vi "Main.vi"() -> ()   [LabVIEW 2015]
panel:
  in  "Load Config":bool
  in  "Save Config":bool
  in  "Configuation Path":path
  out "Real Milliseconds per Packet":sgl=50.0
  in  "Apply New Milliseconds":bool
  in  "Milliseconds per Packet":sgl=50.0
  in  "Apply New X Axis":bool
  in  "Number of Seconds Visible":dbl=10.0
  in  "0":T1={"DeviceType"=0, "DeviceID"=0, "PropertyID"=0, "UpdateProperty"=FALSE, "Current Value"=0.0, "Y-Axis"=0, "Plot Color"=16777215, "Point Color"=16777216} {"DeviceType" items=["Talon", "DIO", "RoboRIO"]; "Y-Axis" items=["Red Axis", "Blue Axis", "Green Axis", "Yellow Axis"]}
  in  "Plot":T2={"0"={"DeviceType"=0, "DeviceID"=0, "PropertyID"=0, "UpdateProperty"=FALSE, "Current Value"=0.0, "Y-Axis"=0, "Plot Color"=16777215, "Point Color"=16777216}, "0 2"={"DeviceType"=0, "DeviceID"=0, "PropertyID"=0, "UpdateProperty"=FALSE, "Current Value"=0.0, "Y-Axis"=0, "Plot Color"=16777215, "Point Color"=16777216}, "0 3"={"DeviceType"=0, "DeviceID"=0, "PropertyID"=0, "UpdateProperty"=FALSE, "Current Value"=0.0, "Y-Axis"=0, "Plot Color"=16777215, "Point Color"=16777216}, "0 4"={"DeviceType"=0, "DeviceID"=0, "PropertyID"=0, "UpdateProperty"=FALSE, "Current Value"=0.0, "Y-Axis"=0, "Plot Color"=16777215, "Point Color"=16777216}, "0 5"={"DeviceType"=0, "DeviceID"=0, "PropertyID"=0, "UpdateProperty"=FALSE, "Current Value"=0.0, "Y-Axis"=0, "Plot Color"=16777215, "Point Color"=16777216}, "0 6"={"DeviceType"=0, "DeviceID"=0, "PropertyID"=0, "UpdateProperty"=FALSE, "Current Value"=0.0, "Y-Axis"=0, "Plot Color"=16777215, "Point Color"=16777216}, "0 7"={"DeviceType"=0, "DeviceID"=0, "PropertyID"=0, "UpdateProperty"=FALSE, "Current Value"=0.0, "Y-Axis"=0, "Plot Color"=16777215, "Point Color"=16777216}, "0 8"={"DeviceType"=0, "DeviceID"=0, "PropertyID"=0, "UpdateProperty"=FALSE, "Current Value"=0.0, "Y-Axis"=0, "Plot Color"=16777215, "Point Color"=16777216}, "0 9"={"DeviceType"=0, "DeviceID"=0, "PropertyID"=0, "UpdateProperty"=FALSE, "Current Value"=0.0, "Y-Axis"=0, "Plot Color"=16777215, "Point Color"=16777216}, "0 10"={"DeviceType"=0, "DeviceID"=0, "PropertyID"=0, "UpdateProperty"=FALSE, "Current Value"=0.0, "Y-Axis"=0, "Plot Color"=16777215, "Point Color"=16777216}, "0 11"={"DeviceType"=0, "DeviceID"=0, "PropertyID"=0, "UpdateProperty"=FALSE, "Current Value"=0.0, "Y-Axis"=0, "Plot Color"=16777215, "Point Color"=16777216}, "0 12"={"DeviceType"=0, "DeviceID"=0, "PropertyID"=0, "UpdateProperty"=FALSE, "Current Value"=0.0, "Y-Axis"=0, "Plot Color"=16777215, "Point Color"=16777216}, "0 13"={"DeviceType"=0, "DeviceID"=0, "PropertyID"=0, "UpdateProperty"=FALSE, "Current Value"=0.0, "Y-Axis"=0, "Plot Color"=16777215, "Point Color"=16777216}, "0 14"={"DeviceType"=0, "DeviceID"=0, "PropertyID"=0, "UpdateProperty"=FALSE, "Current Value"=0.0, "Y-Axis"=0, "Plot Color"=16777215, "Point Color"=16777216}, "0 15"={"DeviceType"=0, "DeviceID"=0, "PropertyID"=0, "UpdateProperty"=FALSE, "Current Value"=0.0, "Y-Axis"=0, "Plot Color"=16777215, "Point Color"=16777216}, "0 16"={"DeviceType"=0, "DeviceID"=0, "PropertyID"=0, "UpdateProperty"=FALSE, "Current Value"=0.0, "Y-Axis"=0, "Plot Color"=16777215, "Point Color"=16777216}} {"0 16"."DeviceID" items=["2"]; "0 16"."PropertyID" items=["SetValue", "OutputVoltage", "OutputCurrent", "EncoderPosition", "EncoderVelocity", "CTR_Absolute_Pos", "ControlLoop_Error", "I Accum", "Supply Voltage", "Forward Hard Limit", "Reverse Hard Limit", "Forward Soft Limit", "Reverse Soft Limit", "Analog In"]; "0 16"."DeviceType" items=["Talon", "DIO", "RoboRIO"]; "0 16"."Y-Axis" items=["Red Axis", "Blue Axis", "Green Axis", "Yellow Axis"]; "0 15"."DeviceID" items=["2"]; "0 15"."PropertyID" items=["SetValue", "OutputVoltage", "OutputCurrent", "EncoderPosition", "EncoderVelocity", "CTR_Absolute_Pos", "ControlLoop_Error", "I Accum", "Supply Voltage", "Forward Hard Limit", "Reverse Hard Limit", "Forward Soft Limit", "Reverse Soft Limit", "Analog In"]; "0 15"."DeviceType" items=["Talon", "DIO", "RoboRIO"]; "0 15"."Y-Axis" items=["Red Axis", "Blue Axis", "Green Axis", "Yellow Axis"]; "0 14"."DeviceID" items=["2"]; "0 14"."PropertyID" items=["SetValue", "OutputVoltage", "OutputCurrent", "EncoderPosition", "EncoderVelocity", "CTR_Absolute_Pos", "ControlLoop_Error", "I Accum", "Supply Voltage", "Forward Hard Limit", "Reverse Hard Limit", "Forward Soft Limit", "Reverse Soft Limit", "Analog In"]; "0 14"."DeviceType" items=["Talon", "DIO", "RoboRIO"]; "0 14"."Y-Axis" items=["Red Axis", "Blue Axis", "Green Axis", "Yellow Axis"]; "0 13"."DeviceID" items=["2"]; "0 13"."PropertyID" items=["SetValue", "OutputVoltage", "OutputCurrent", "EncoderPosition", "EncoderVelocity", "CTR_Absolute_Pos", "ControlLoop_Error", "I Accum", "Supply Voltage", "Forward Hard Limit", "Reverse Hard Limit", "Forward Soft Limit", "Reverse Soft Limit", "Analog In"]; "0 13"."DeviceType" items=["Talon", "DIO", "RoboRIO"]; "0 13"."Y-Axis" items=["Red Axis", "Blue Axis", "Green Axis", "Yellow Axis"]; "0 12"."DeviceID" items=["2"]; "0 12"."PropertyID" items=["SetValue", "OutputVoltage", "OutputCurrent", "EncoderPosition", "EncoderVelocity", "CTR_Absolute_Pos", "ControlLoop_Error", "I Accum", "Supply Voltage", "Forward Hard Limit", "Reverse Hard Limit", "Forward Soft Limit", "Reverse Soft Limit", "Analog In"]; "0 12"."DeviceType" items=["Talon", "DIO", "RoboRIO"]; "0 12"."Y-Axis" items=["Red Axis", "Blue Axis", "Green Axis", "Yellow Axis"]; "0 11"."DeviceID" items=["2"]; "0 11"."PropertyID" items=["SetValue", "OutputVoltage", "OutputCurrent", "EncoderPosition", "EncoderVelocity", "CTR_Absolute_Pos", "ControlLoop_Error", "I Accum", "Supply Voltage", "Forward Hard Limit", "Reverse Hard Limit", "Forward Soft Limit", "Reverse Soft Limit", "Analog In"]; "0 11"."DeviceType" items=["Talon", "DIO", "RoboRIO"]; "0 11"."Y-Axis" items=["Red Axis", "Blue Axis", "Green Axis", "Yellow Axis"]; "0 10"."DeviceID" items=["2"]; "0 10"."PropertyID" items=["SetValue", "OutputVoltage", "OutputCurrent", "EncoderPosition", "EncoderVelocity", "CTR_Absolute_Pos", "ControlLoop_Error", "I Accum", "Supply Voltage", "Forward Hard Limit", "Reverse Hard Limit", "Forward Soft Limit", "Reverse Soft Limit", "Analog In"]; "0 10"."DeviceType" items=["Talon", "DIO", "RoboRIO"]; "0 10"."Y-Axis" items=["Red Axis", "Blue Axis", "Green Axis", "Yellow Axis"]; "0 9"."DeviceID" items=["2"]; "0 9"."PropertyID" items=["SetValue", "OutputVoltage", "OutputCurrent", "EncoderPosition", "EncoderVelocity", "CTR_Absolute_Pos", "ControlLoop_Error", "I Accum", "Supply Voltage", "Forward Hard Limit", "Reverse Hard Limit", "Forward Soft Limit", "Reverse Soft Limit", "Analog In"]; "0 9"."DeviceType" items=["Talon", "DIO", "RoboRIO"]; "0 9"."Y-Axis" items=["Red Axis", "Blue Axis", "Green Axis", "Yellow Axis"]; "0 8"."DeviceID" items=["2"]; "0 8"."PropertyID" items=["SetValue", "OutputVoltage", "OutputCurrent", "EncoderPosition", "EncoderVelocity", "CTR_Absolute_Pos", "ControlLoop_Error", "I Accum", "Supply Voltage", "Forward Hard Limit", "Reverse Hard Limit", "Forward Soft Limit", "Reverse Soft Limit", "Analog In"]; "0 8"."DeviceType" items=["Talon", "DIO", "RoboRIO"]; "0 8"."Y-Axis" items=["Red Axis", "Blue Axis", "Green Axis", "Yellow Axis"]; "0 7"."DeviceID" items=["2"]; "0 7"."PropertyID" items=["SetValue", "OutputVoltage", "OutputCurrent", "EncoderPosition", "EncoderVelocity", "CTR_Absolute_Pos", "ControlLoop_Error", "I Accum", "Supply Voltage", "Forward Hard Limit", "Reverse Hard Limit", "Forward Soft Limit", "Reverse Soft Limit", "Analog In"]; "0 7"."DeviceType" items=["Talon", "DIO", "RoboRIO"]; "0 7"."Y-Axis" items=["Red Axis", "Blue Axis", "Green Axis", "Yellow Axis"]; "0 6"."DeviceID" items=["2"]; "0 6"."PropertyID" items=["SetValue", "OutputVoltage", "OutputCurrent", "EncoderPosition", "EncoderVelocity", "CTR_Absolute_Pos", "ControlLoop_Error", "I Accum", "Supply Voltage", "Forward Hard Limit", "Reverse Hard Limit", "Forward Soft Limit", "Reverse Soft Limit", "Analog In"]; "0 6"."DeviceType" items=["Talon", "DIO", "RoboRIO"]; "0 6"."Y-Axis" items=["Red Axis", "Blue Axis", "Green Axis", "Yellow Axis"]; "0 5"."DeviceID" items=["2"]; "0 5"."PropertyID" items=["SetValue", "OutputVoltage", "OutputCurrent", "EncoderPosition", "EncoderVelocity", "CTR_Absolute_Pos", "ControlLoop_Error", "I Accum", "Supply Voltage", "Forward Hard Limit", "Reverse Hard Limit", "Forward Soft Limit", "Reverse Soft Limit", "Analog In"]; "0 5"."DeviceType" items=["Talon", "DIO", "RoboRIO"]; "0 5"."Y-Axis" items=["Red Axis", "Blue Axis", "Green Axis", "Yellow Axis"]; "0 4"."DeviceID" items=["2"]; "0 4"."PropertyID" items=["SetValue", "OutputVoltage", "OutputCurrent", "EncoderPosition", "EncoderVelocity", "CTR_Absolute_Pos", "ControlLoop_Error", "I Accum", "Supply Voltage", "Forward Hard Limit", "Reverse Hard Limit", "Forward Soft Limit", "Reverse Soft Limit", "Analog In"]; "0 4"."DeviceType" items=["Talon", "DIO", "RoboRIO"]; "0 4"."Y-Axis" items=["Red Axis", "Blue Axis", "Green Axis", "Yellow Axis"]; "0 3"."DeviceID" items=["2"]; "0 3"."PropertyID" items=["SetValue", "OutputVoltage", "OutputCurrent", "EncoderPosition", "EncoderVelocity", "CTR_Absolute_Pos", "ControlLoop_Error", "I Accum", "Supply Voltage", "Forward Hard Limit", "Reverse Hard Limit", "Forward Soft Limit", "Reverse Soft Limit", "Analog In"]; "0 3"."DeviceType" items=["Talon", "DIO", "RoboRIO"]; "0 3"."Y-Axis" items=["Red Axis", "Blue Axis", "Green Axis", "Yellow Axis"]; "0 2"."DeviceID" items=["0"]; "0 2"."PropertyID" items=["PacketCounter", "Milliseconds Per Packet", "CPU Load"]; "0 2"."DeviceType" items=["Talon", "DIO", "RoboRIO"]; "0 2"."Y-Axis" items=["Red Axis", "Blue Axis", "Green Axis", "Yellow Axis"]; "0"."DeviceID" items=["0"]; "0"."PropertyID" items=["Value"]; "0"."DeviceType" items=["Talon", "DIO", "RoboRIO"]; "0"."Y-Axis" items=["Red Axis", "Blue Axis", "Green Axis", "Yellow Axis"]}
  in  "Stop Data":bool
  out "Raw Data Packet":string
  out "Waveform chart":waveform(dbl)[](graph)=[{"t0"=timestamp(3553447770.6895175 s since 1904-01-01), "dt"=1.0, "Y"=[0.0]}, {"t0"=timestamp(3553447770.6895175 s since 1904-01-01), "dt"=1.0, "Y"=[nan]}, {"t0"=timestamp(3553447770.6895175 s since 1904-01-01), "dt"=1.0, "Y"=[nan]}, {"t0"=timestamp(3553447770.6895175 s since 1904-01-01), "dt"=1.0, "Y"=[nan]}, {"t0"=timestamp(3553447770.6895175 s since 1904-01-01), "dt"=1.0, "Y"=[nan]}, {"t0"=timestamp(3553447770.6895175 s since 1904-01-01), "dt"=1.0, "Y"=[nan]}, {"t0"=timestamp(3553447770.6895175 s since 1904-01-01), "dt"=1.0, "Y"=[nan]}, {"t0"=timestamp(3553447770.6895175 s since 1904-01-01), "dt"=1.0, "Y"=[nan]}, {"t0"=timestamp(3553447770.6895175 s since 1904-01-01), "dt"=1.0, "Y"=[nan]}, {"t0"=timestamp(3553447770.6895175 s since 1904-01-01), "dt"=1.0, "Y"=[nan]}, {"t0"=timestamp(3553447770.6895175 s since 1904-01-01), "dt"=1.0, "Y"=[nan]}, {"t0"=timestamp(3553447770.6895175 s since 1904-01-01), "dt"=1.0, "Y"=[nan]}, {"t0"=timestamp(3553447770.6895175 s since 1904-01-01), "dt"=1.0, "Y"=[nan]}, {"t0"=timestamp(3553447770.6895175 s since 1904-01-01), "dt"=1.0, "Y"=[nan]}, {"t0"=timestamp(3553447770.6895175 s since 1904-01-01), "dt"=1.0, "Y"=[nan]}, {"t0"=timestamp(3553447770.6895175 s since 1904-01-01), "dt"=1.0, "Y"=[nan]}]
  out "UDPRecv Error":errorcluster={"status"=TRUE, "code"=56, "source"="UDP Read in Main.vi"}
  out "Status":string
  out "DeviceIDs arranged by Type":u8[][](array[numeric])
  # "Grapher v6"
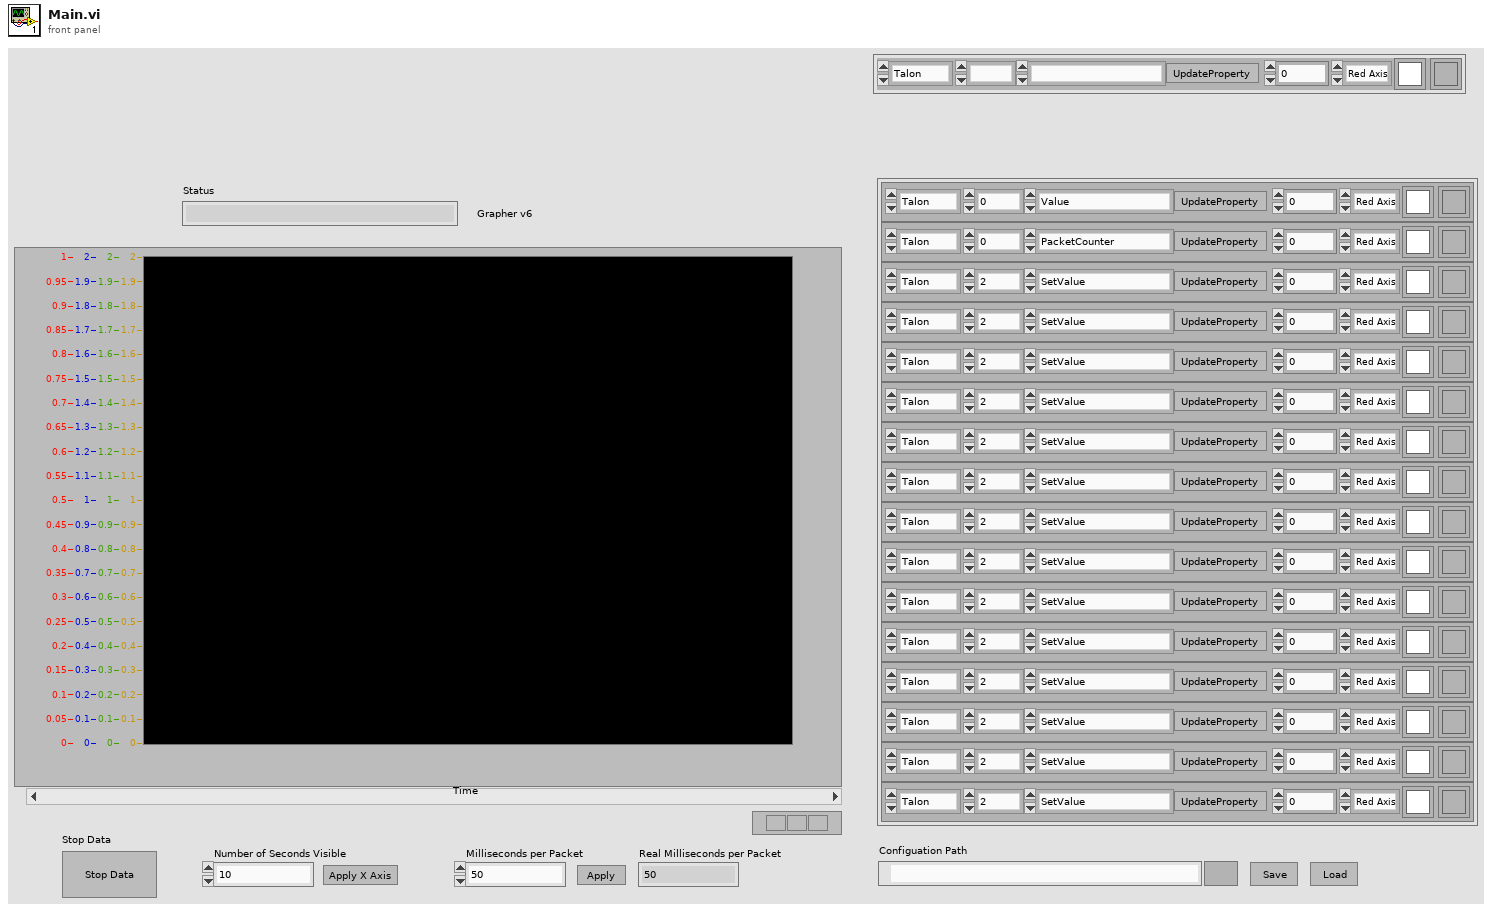
[diagram p1: front panel]
types:
  T1 = cluster{"DeviceType":u8, "DeviceID":u8, "PropertyID":u8, "UpdateProperty":bool, "Current Value":dbl, "Y-Axis":u16, "Plot Color":u32, "Point Color":u32}
  T2 = cluster{"0":cluster{"DeviceType":u8, "DeviceID":u8, "PropertyID":u8, "UpdateProperty":bool, "Current Value":dbl, "Y-Axis":u16, "Plot Color":u32, "Point Color":u32}, "0 2":cluster{"DeviceType":u8, "DeviceID":u8, "PropertyID":u8, "UpdateProperty":bool, "Current Value":dbl, "Y-Axis":u16, "Plot Color":u32, "Point Color":u32}, "0 3":cluster{"DeviceType":u8, "DeviceID":u8, "PropertyID":u8, "UpdateProperty":bool, "Current Value":dbl, "Y-Axis":u16, "Plot Color":u32, "Point Color":u32}, "0 4":cluster{"DeviceType":u8, "DeviceID":u8, "PropertyID":u8, "UpdateProperty":bool, "Current Value":dbl, "Y-Axis":u16, "Plot Color":u32, "Point Color":u32}, "0 5":cluster{"DeviceType":u8, "DeviceID":u8, "PropertyID":u8, "UpdateProperty":bool, "Current Value":dbl, "Y-Axis":u16, "Plot Color":u32, "Point Color":u32}, "0 6":cluster{"DeviceType":u8, "DeviceID":u8, "PropertyID":u8, "UpdateProperty":bool, "Current Value":dbl, "Y-Axis":u16, "Plot Color":u32, "Point Color":u32}, "0 7":cluster{"DeviceType":u8, "DeviceID":u8, "PropertyID":u8, "UpdateProperty":bool, "Current Value":dbl, "Y-Axis":u16, "Plot Color":u32, "Point Color":u32}, "0 8":cluster{"DeviceType":u8, "DeviceID":u8, "PropertyID":u8, "UpdateProperty":bool, "Current Value":dbl, "Y-Axis":u16, "Plot Color":u32, "Point Color":u32}, "0 9":cluster{"DeviceType":u8, "DeviceID":u8, "PropertyID":u8, "UpdateProperty":bool, "Current Value":dbl, "Y-Axis":u16, "Plot Color":u32, "Point Color":u32}, "0 10":cluster{"DeviceType":u8, "DeviceID":u8, "PropertyID":u8, "UpdateProperty":bool, "Current Value":dbl, "Y-Axis":u16, "Plot Color":u32, "Point Color":u32}, "0 11":cluster{"DeviceType":u8, "DeviceID":u8, "PropertyID":u8, "UpdateProperty":bool, "Current Value":dbl, "Y-Axis":u16, "Plot Color":u32, "Point Color":u32}, "0 12":cluster{"DeviceType":u8, "DeviceID":u8, "PropertyID":u8, "UpdateProperty":bool, "Current Value":dbl, "Y-Axis":u16, "Plot Color":u32, "Point Color":u32}, "0 13":cluster{"DeviceType":u8, "DeviceID":u8, "PropertyID":u8, "UpdateProperty":bool, "Current Value":dbl, "Y-Axis":u16, "Plot Color":u32, "Point Color":u32}, "0 14":cluster{"DeviceType":u8, "DeviceID":u8, "PropertyID":u8, "UpdateProperty":bool, "Current Value":dbl, "Y-Axis":u16, "Plot Color":u32, "Point Color":u32}, "0 15":cluster{"DeviceType":u8, "DeviceID":u8, "PropertyID":u8, "UpdateProperty":bool, "Current Value":dbl, "Y-Axis":u16, "Plot Color":u32, "Point Color":u32}, "0 16":cluster{"DeviceType":u8, "DeviceID":u8, "PropertyID":u8, "UpdateProperty":bool, "Current Value":dbl, "Y-Axis":u16, "Plot Color":u32, "Point Color":u32}}
  T3 = cluster{"Scales":cluster{"Max":dbl, "Min":dbl}[]}
  T4 = enum8{"DeviceListRequest", "DeviceList", "UpdateSubscription", "SubscriptionData"}
  T5 = cluster{enum8{"DeviceListRequest", "DeviceList", "UpdateSubscription", "SubscriptionData"}, u8, "DeviceType":u8, u8, "PropertyID":u8}
  T6 = enum16{"open", "replace", "create", "open or create", "replace or create", "replace or create with confirmation"}
  T7 = enum8{"DeviceListRequest", "DeviceList", "UpdateSubscription", "SubscriptionData", "ChangeUpdateRate"}
  T8 = cluster{"YScale.Maximum":dbl, "YScale.Minimum":dbl}
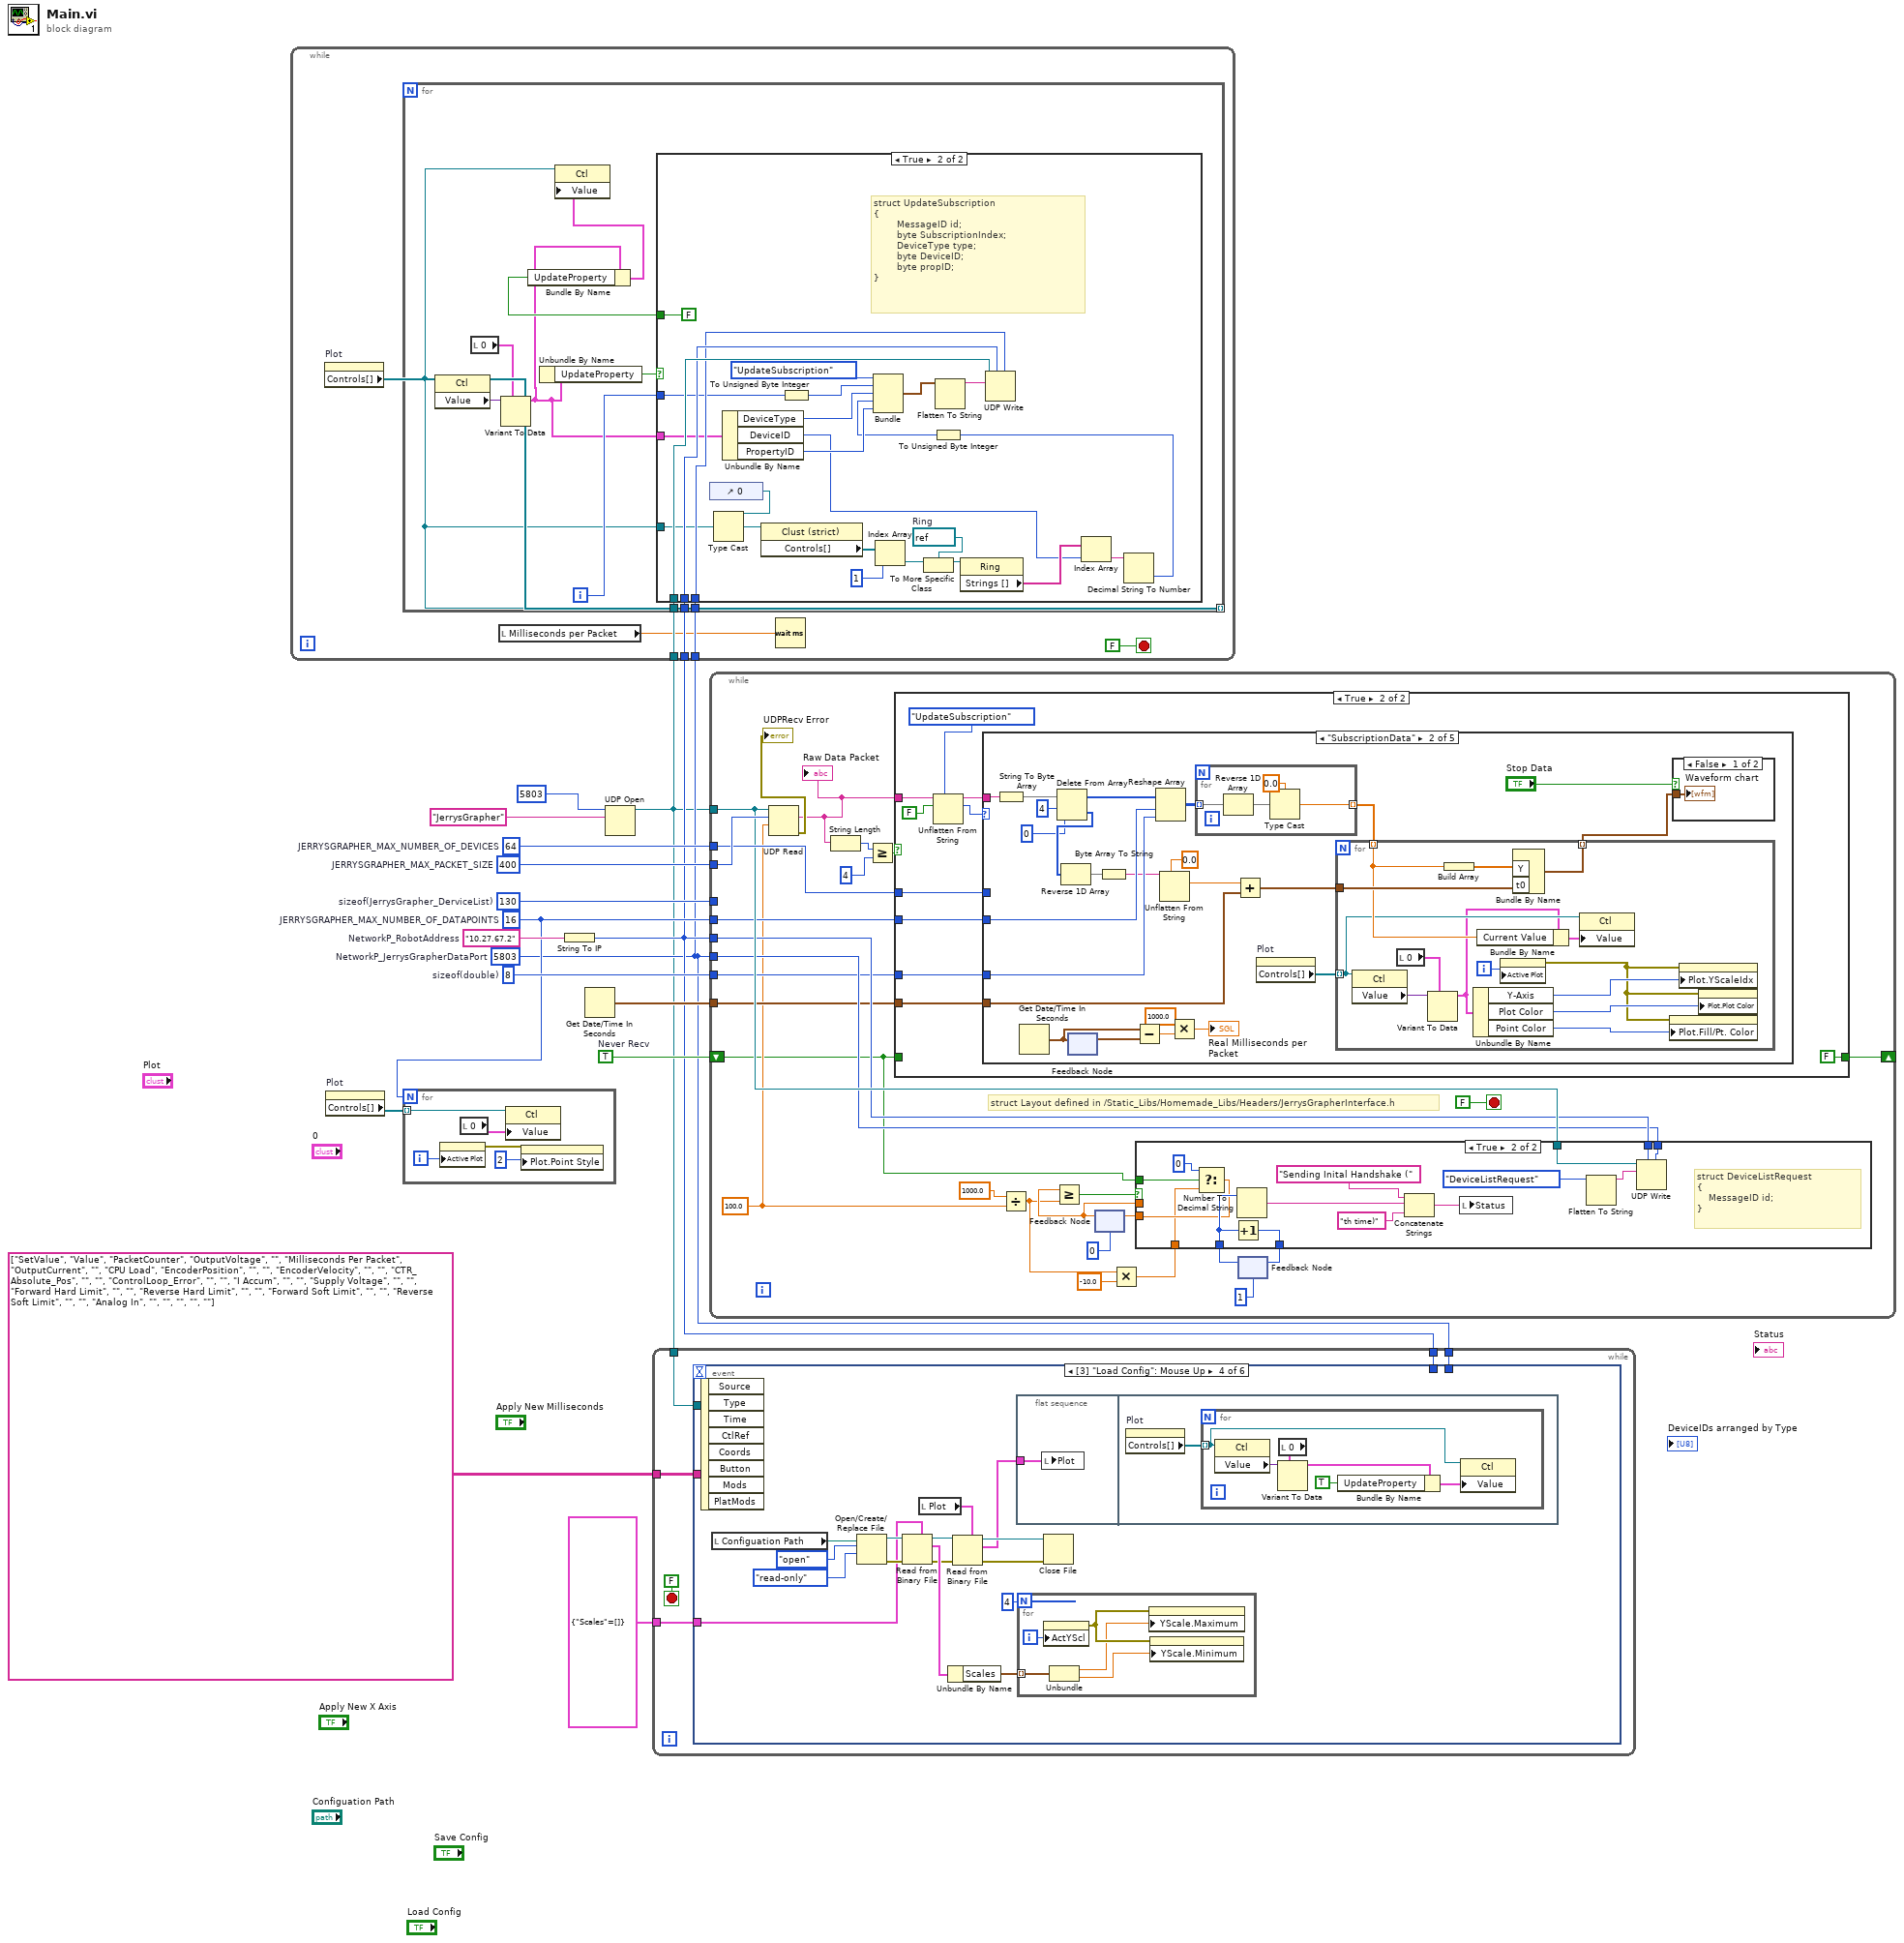
[diagram p0: block diagram]
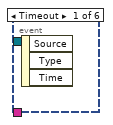
[diagram p3: hidden frame]
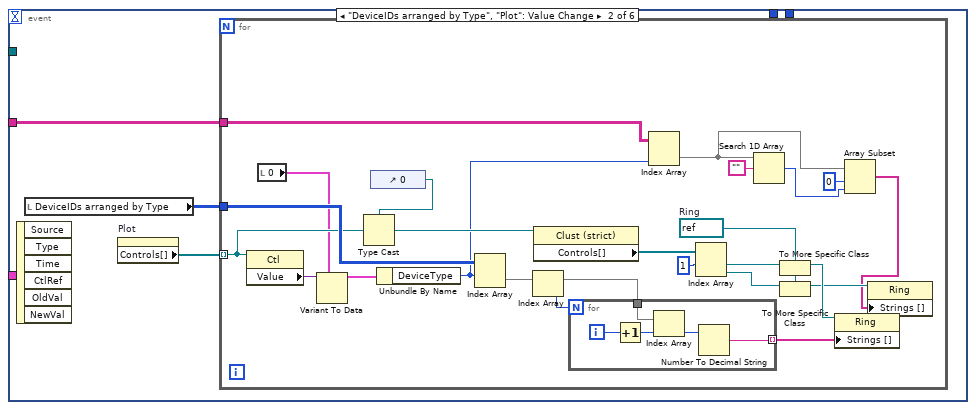
[diagram p4: hidden frame]
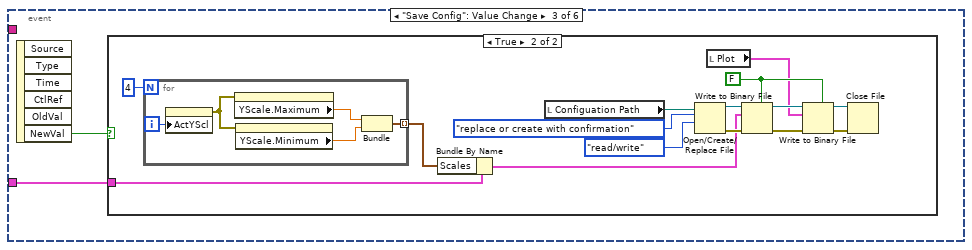
[diagram p5: hidden frame]
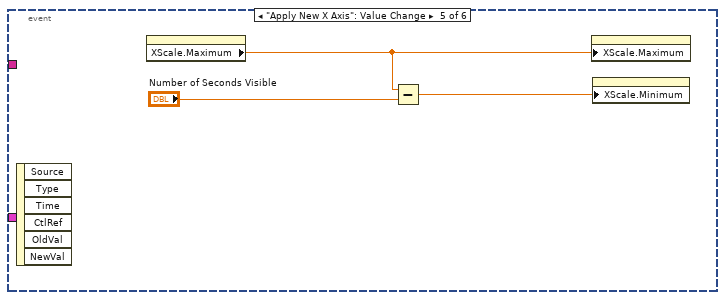
[diagram p7: hidden frame]
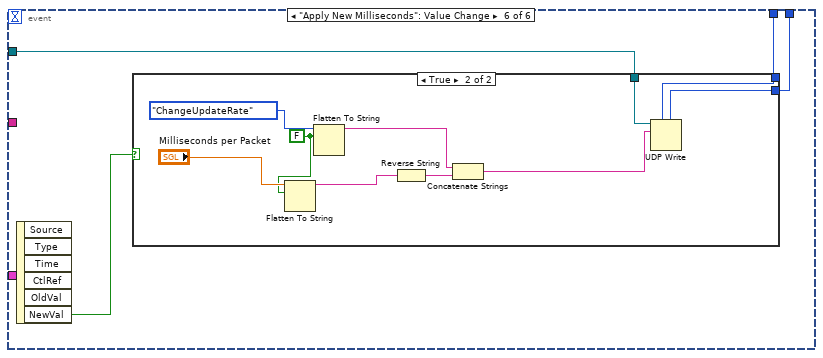
[diagram p8: hidden frame]
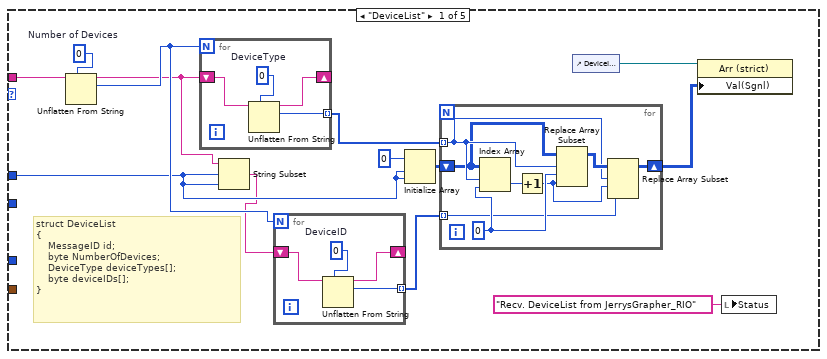
[diagram p11: hidden frame]
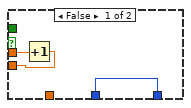
[diagram p16: hidden frame]
diagram:
  w9 = 8  # sizeof(double)
  w8 = 16  # JERRYSGRAPHER_MAX_NUMBER_OF_DATAPOINTS
  w3 = 5803  # NetworkP_JerrysGrapherDataPort
  w10 = 64  # JERRYSGRAPHER_MAX_NUMBER_OF_DEVICES
  w12 = 400  # JERRYSGRAPHER_MAX_PACKET_SIZE
  w13 = TRUE  # Never Recv
  w14 = "10.27.67.2"  # NetworkP_RobotAddress
  w11 = 130  # sizeof(JerrysGrapher_DerviceList)
  n1 = property on="Plot" class="Clust (strict)"() -> ("Controls[]"=w6:refnum<vi>[])  [unwired: 2 in, 2 out]
  n2 = for {
    N: w8 -> [_]
    tunnel: w6 -> [w21] mode=indexing
    i -> [w17]
    n3 = property on="Waveform chart" class="WFChart (strict)"("Active Plot"=w17) -> (error out=w19:errorcluster)  [unwired: 2 in, 1 out]
    n4 = local read "0"() -> (w20:T1)
    n5 = property class="Ctl"(reference=w21, "Value"=w20) -> ()  [unwired: 1 in, 2 out]
    n6 = property on="Waveform chart" class="WFChart (strict)"(error in=w19, "Plot.Point Style"=u8 2) -> ()  [unwired: 1 in, 2 out]
  }
  n7 = String To IP(1:w14) -> (0:w4:u32)
  n8 = Get Date/Time In Seconds() -> (seconds since 1Jan1904=w7:timestamp)
  n9 = UDP Open(10:"JerrysGrapher" ("service name"), 11:u16 5803 ("port")) -> (port=w2:refnum<k16>)  [unwired: 3 in, 2 out]
  n10 = while {
    tunnel: w4 -> [w25]
    tunnel: w2 -> [w26]
    tunnel: w3 -> [w24]
    stop <- FALSE stop-if-true
    n11 = property on="Plot" class="Clust (strict)"() -> ("Controls[]"=w23:refnum<vi>[])  [unwired: 2 in, 2 out]
    n12 = for {
      tunnel: w26 -> [w38]
      tunnel: w25 -> [w37]
      tunnel: w24 -> [w36]
      tunnel: w23 -> [w28] mode=indexing
      i -> [w35]
      n13 = property class="Ctl"(reference=w28) -> ("Value"=w34:variant)  [unwired: 1 in, 2 out]
      n14 = local read "0"() -> (w33:T1)
      n15 = Variant To Data(type=w33, Variant=w34) -> (data=w29:T1)  [unwired: 1 in, 1 out]
      n16 = Unbundle By Name(w29) -> ("UpdateProperty"=w32:bool)
      n17 = case shown="True" w32 {
        selector: w32 -> [w39 _]
        tunnel: w38 -> [_ w62]
        tunnel: w37 -> [_ w59]
        tunnel: w36 -> [_ w58]
        tunnel: w35 -> [_ w55]
        tunnel: [w39 FALSE] -> w31
        tunnel: w29 -> [_ w53]
        tunnel: w28 -> [_ w52]
        frame False {
        }
        frame True {
          w46 = refnum<vi> refnum  # Ring
          # "struct UpdateSubscription\n{\n        MessageID id;\n        byte SubscriptionIndex;\n        DeviceType type;\n        byte DeviceID;\n        byte propID;\n}"
          n18 = control-ref of="0"() -> (w50:refnum<vi>)
          n19 = Type Cast(type=w50, x=w52) -> (*(type *) &x=w51:refnum<vi>)
          n20 = Unbundle By Name(w53) -> ("DeviceType"=w64:u8, "DeviceID"=w43:u8, "PropertyID"=w63:u8)
          n21 = property class="Clust (strict)"(reference=w51) -> ("Controls[]"=w49:refnum<vi>[])  [unwired: 1 in, 2 out]
          n22 = To Unsigned Byte Integer(number=w55) -> (unsigned 8bit integer=w56:u8)
          n23 = Index Array(array=w49, index=1) -> (element=w47:refnum<vi>)
          n24 = To More Specific Class(target class=w46, reference=w47) -> (specific class reference=w45:refnum<vi>)  [unwired: 1 in, 1 out]
          n25 = property class="Ring"(reference=w45) -> ("Strings []"=w44:string[])  [unwired: 1 in, 2 out]
          n26 = Index Array(array=w44, index=w43) -> (element=w42:string)
          n27 = Decimal String To Number(string=w42) -> (number=w41:i32)  [unwired: 2 in, 1 out]
          n28 = To Unsigned Byte Integer(number=w41) -> (unsigned 8bit integer=w40:u8)
          n29 = Bundle(T4."UpdateSubscription", w56, "DeviceType"=w64, w40, "PropertyID"=w63) -> (w61:T5)  [unwired: 1 in]
          n30 = Flatten To String(anything=w61) -> (data string=w60:string)  [unwired: 3 in, 2 out]
          n31 = UDP Write(address=w59, port or service name=w58, connection ID=w62, data in=w60) -> ()  [unwired: 2 in, 2 out]
        }
      }
      n32 = Bundle By Name(cluster=w29, "UpdateProperty"=w31) -> (w30:T1)
      n33 = property class="Ctl"(reference=w28, "Value"=w30) -> ()  [unwired: 1 in, 2 out]
    }
    n34 = local read "Milliseconds per Packet"() -> (w22:sgl)
    n35 = Wait (ms)(milliseconds to wait=w22) -> ()  [unwired: 1 out]
  }
  n36 = while {
    tunnel: string[][] [["SetValue", "Value", "PacketCounter"], ["OutputVoltage", "", "Milliseconds Per Packet"], ["OutputCurrent", "", "CPU Load"], ["EncoderPosition", "", ""], ["EncoderVelocity", "", ""], ["CTR_Absolute_Pos", "", ""], ["ControlLoop_Error", "", ""], ["I Accum", "", ""], ["Supply Voltage", "", ""], ["Forward Hard Limit", "", ""], ["Reverse Hard Limit", "", ""], ["Forward Soft Limit", "", ""], ["Reverse Soft Limit", "", ""], ["Analog In", "", ""], ["", "", ""]] -> [w69]
    tunnel: w4 -> [w68]
    tunnel: w3 -> [w67]
    tunnel: w2 -> [w66]
    tunnel: T3 {"Scales"=[]} -> [w65]
    stop <- FALSE stop-if-true
    n37 = event shown="[3] \"Load Config\": Mouse Up" {
      selector: _ -> [_ _ _ _ _ _]
      dyn-events: _ -> [_ _ _ _ _ _]
      timeout: _ -> [_ _ _ _ _ _]
      tunnel: w69 -> [_ w71 _ _ _ _]
      tunnel: w68 -> [_ _ _ _ _ w159]
      tunnel: w67 -> [_ _ _ _ _ w158]
      tunnel: w66 -> [_ _ _ _ _ w157]
      tunnel: w65 -> [_ _ w104 w133 _ _]
      event Timeout {
        n38 = event-data() -> ()  [unwired: 1 in, 3 out]
      }
      event "DeviceIDs arranged by Type", "Plot": Value Change {
        n39 = event-data() -> ()  [unwired: 1 in, 6 out]
        n40 = local read "DeviceIDs arranged by Type"() -> (w73:u8[][])
        n41 = property on="Plot" class="Clust (strict)"() -> ("Controls[]"=w72:refnum<vi>[])  [unwired: 2 in, 2 out]
        n42 = for {
          tunnel: w73 -> [w97]
          tunnel: w72 -> [w91] mode=indexing
          tunnel: w71 -> [w79]
          w82 = refnum<vi> refnum  # Ring
          n43 = property class="Ctl"(reference=w91) -> ("Value"=w93:variant)  [unwired: 1 in, 2 out]
          n44 = local read "0"() -> (w84:T1)
          n45 = Variant To Data(type=w84, Variant=w93) -> (data=w92:T1)  [unwired: 1 in, 1 out]
          n46 = control-ref of="0"() -> (w85:refnum<vi>)
          n47 = Type Cast(type=w85, x=w91) -> (*(type *) &x=w86:refnum<vi>)
          n48 = Unbundle By Name(w92) -> ("DeviceType"=w80:u8)
          n49 = Index Array(array=w97, index (row)=w80) -> (element=w95:u8[])  [unwired: 1 in]
          n50 = Index Array(array=w95) -> (element=w96:u8)  [unwired: 1 in]
          n51 = property class="Clust (strict)"(reference=w86) -> ("Controls[]"=w90:refnum<vi>[])  [unwired: 1 in, 2 out]
          n52 = for {
            N: w96 -> [_]
            tunnel: w95 -> [w102]
            tunnel: [w98] -> w94 mode=indexing
            i -> [w101]
            n53 = Increment(x=w101) -> (x+1=w100:i32)
            n54 = Index Array(array=w102, index=w100) -> (element=w99:u8)
            n55 = Number To Decimal String(number=w99) -> (decimal integer string=w98:string)  [unwired: 1 in]
          }
          n56 = Index Array(array=w79, index (col)=w80) -> (element=w77:string[])  [unwired: 1 in]
          n57 = Index Array(array=w90, index #1=1 ("index")) -> (element #1=w88:refnum<vi>, element #2=w83:refnum<vi>)  [unwired: 1 in]
          n58 = Search 1D Array(1D array=w77, element="") -> (index of element=w75:i32)  [unwired: 1 in]
          n59 = To More Specific Class(target class=w82, reference=w88) -> (specific class reference=w87:refnum<vi>)  [unwired: 1 in, 1 out]
          n60 = To More Specific Class(target class=w82, reference=w83) -> (specific class reference=w81:refnum<vi>)  [unwired: 1 in, 1 out]
          n61 = property class="Ring"(reference=w87, "Strings []"=w94) -> ()  [unwired: 1 in, 2 out]
          n62 = Array Subset(array=w77, index=0, length=w75) -> (w74:string[])
          n63 = property class="Ring"(reference=w81, "Strings []"=w74) -> ()  [unwired: 1 in, 2 out]
        }
      }
      event "Save Config": Value Change {
        n64 = event-data() -> ("NewVal"=w103:bool)  [unwired: 1 in, 5 out]
        n65 = case shown="True" w103 {
          tunnel: w104 -> [_ w112]
          frame False {
          }
          frame True {
            w108 = FALSE ("prepend array or string size? (T)")
            n66 = for {
              N: 4 -> [_]
              tunnel: [w120] -> w113 mode=indexing
              i -> [w123]
              n67 = property on="Waveform chart" class="WFChart (strict)"("ActYScl"=w123) -> (error out=w124:errorcluster)  [unwired: 2 in, 1 out]
              n68 = property on="Waveform chart" class="WFChart (strict)"(error in=w124) -> ("YScale.Maximum"=w122:dbl)  [unwired: 1 in, 2 out]
              n69 = property on="Waveform chart" class="WFChart (strict)"(error in=w124) -> ("YScale.Minimum"=w121:dbl)  [unwired: 1 in, 2 out]
              n70 = Bundle("YScale.Maximum"=w122, "YScale.Minimum"=w121) -> (w120:T8)  [unwired: 1 in]
            }
            n71 = Bundle By Name(cluster=w112, "Scales"=w113) -> (w111:T3)
            n72 = local read "Configuation Path"() -> (w119:path)
            n73 = Open/Create/Replace File(file path (use dialog)=w119, operation (0:open)=T6."replace or create with confirmation", access (0:read/write)=enum16{"read/write", "read-only", "write-only"}."read/write") -> (refnum out=w116:refnum<file>, error out=w115:errorcluster)  [unwired: 3 in, 1 out]
            n74 = local read "Plot"() -> (w105:T2)
            n75 = Write to Binary File(file (use dialog)=w116, data=w111, error in=w115, 5:w108) -> (refnum out=w109:refnum<file>, error out=w110:errorcluster)  [unwired: 2 in, 1 out]
            n76 = Write to Binary File(file (use dialog)=w109, data=w105, error in=w110, 5:w108) -> (refnum out=w107:refnum<file>, error out=w106:errorcluster)  [unwired: 2 in, 1 out]
            n77 = Close File(refnum=w107, error in=w106) -> ()  [unwired: 2 out]
          }
        }
      }
      event "Load Config": Mouse Up {
        n78 = event-data() -> ()  [unwired: 1 in, 8 out]
        n79 = local read "Configuation Path"() -> (w139:path)
        n80 = Open/Create/Replace File(file path (use dialog)=w139, operation (0:open)=T6."open", access (0:read/write)=enum16{"read/write", "read-only", "write-only"}."read-only") -> (refnum out=w136:refnum<file>, error out=w135:errorcluster)  [unwired: 3 in, 1 out]
        n81 = Read from Binary File(5:w133, 8:w135, 11:w136) -> (0:w130:errorcluster, 2:w132:T3, 3:w129:refnum<file>)  [unwired: 3 in, 1 out]
        n82 = local read "Plot"() -> (w126:T2)
        n83 = Unbundle By Name(w132) -> ("Scales"=w131:cluster{"Max":dbl, "Min":dbl}[])
        n84 = Read from Binary File(5:w126, 8:w130, 11:w129) -> (0:w127:errorcluster, 2:w125:T2, 3:w128:refnum<file>)  [unwired: 3 in, 1 out]
        n85 = flat-sequence {
          tunnel: w125 -> [w140]
          frame #0 {
            n86 = local write "Plot"(w140) -> ()
          }
          frame #1 {
            n87 = property on="Plot" class="Clust (strict)"() -> ("Controls[]"=w141:refnum<vi>[])  [unwired: 2 in, 2 out]
            n88 = for {
              tunnel: w141 -> [w142] mode=indexing
              n89 = property class="Ctl"(reference=w142) -> ("Value"=w147:variant)  [unwired: 1 in, 2 out]
              n90 = local read "0"() -> (w146:T1)
              n91 = Variant To Data(type=w146, Variant=w147) -> (data=w145:T1)  [unwired: 1 in, 1 out]
              n92 = Bundle By Name(cluster=w145, "UpdateProperty"=TRUE) -> (w143:T1)
              n93 = property class="Ctl"(reference=w142, "Value"=w143) -> ()  [unwired: 1 in, 2 out]
            }
          }
        }
        n94 = for {
          N: 4 -> [_]
          tunnel: w131 -> [w150] mode=indexing
          i -> [w151]
          n95 = property on="Waveform chart" class="WFChart (strict)"("ActYScl"=w151) -> (error out=w152:errorcluster)  [unwired: 2 in, 1 out]
          n96 = Unbundle(w150) -> ("Max"=w149:dbl, "Min"=w148:dbl)
          n97 = property on="Waveform chart" class="WFChart (strict)"(error in=w152, "YScale.Maximum"=w149) -> ()  [unwired: 1 in, 2 out]
          n98 = property on="Waveform chart" class="WFChart (strict)"(error in=w152, "YScale.Minimum"=w148) -> ()  [unwired: 1 in, 2 out]
        }
        n99 = Close File(refnum=w128, error in=w127) -> ()  [unwired: 2 out]
      }
      event "Apply New X Axis": Value Change {
        n100 = event-data() -> ()  [unwired: 1 in, 6 out]
        n101 = property on="Waveform chart" class="WFChart (strict)"() -> ("XScale.Maximum"=w153:dbl)  [unwired: 2 in, 2 out]
        n102 = Subtract(x=w153, y="Number of Seconds Visible") -> (x-y=w154:dbl)
        n103 = property on="Waveform chart" class="WFChart (strict)"("XScale.Maximum"=w153) -> ()  [unwired: 2 in, 2 out]
        n104 = property on="Waveform chart" class="WFChart (strict)"("XScale.Minimum"=w154) -> ()  [unwired: 2 in, 2 out]
      }
      event "Apply New Milliseconds": Value Change {
        n105 = event-data() -> ("NewVal"=w156:bool)  [unwired: 1 in, 5 out]
        n106 = case shown="True" w156 {
          tunnel: w159 -> [_ w169]
          tunnel: w158 -> [_ w168]
          tunnel: w157 -> [_ w167]
          frame False {
          }
          frame True {
            w162 = FALSE ("prepend array or string size? (T)")
            n107 = Flatten To String(anything="Milliseconds per Packet", prepend array or string size? (T)=w162) -> (data string=w163:string)  [unwired: 2 in, 2 out]
            n108 = Flatten To String(anything=T7."ChangeUpdateRate", prepend array or string size? (T)=w162) -> (data string=w164:string)  [unwired: 2 in, 2 out]
            n109 = Reverse String(1:w163) -> (0:w160:string)
            n110 = Concatenate Strings(w164, w160) -> (w161:string)
            n111 = UDP Write(address=w169, port or service name=w168, connection ID=w167, data in=w161) -> ()  [unwired: 2 in, 2 out]
          }
        }
      }
    }
  }
  n112 = while {
    shift-right: [w195] -> _
    shift-left: w13 -> [w173]
    tunnel: w2 -> [w183]
    tunnel: w12 -> [w196]
    tunnel: w11 -> [_]
    tunnel: w10 -> [w194]
    tunnel: w4 -> [w182]
    tunnel: w3 -> [w181]
    tunnel: w9 -> [w178]
    tunnel: w8 -> [w177]
    tunnel: w7 -> [w176]
    stop <- FALSE stop-if-true
    w175 = 100.0
    # "struct Layout defined in /Static_Libs/Homemade_Libs/Headers/JerrysGrapherInterface.h"
    n113 = UDP Read(connection ID=w183, max size (548)=w196, timeout ms (25000)=w175) -> (data out=w179:string, error out=→"UDPRecv Error":errorcluster)  [unwired: 1 in, 3 out]
    "Raw Data Packet" <- w179
    n114 = String Length(string=w179) -> (length=w192:i32)
    n115 = Greater Or Equal?(x=w192, y=4) -> (x >= y?=w193:bool)
    n116 = case shown="True" w193 {
      tunnel: [w198 FALSE ("Never Recv")] -> w195
      tunnel: w194 -> [_ w208]
      tunnel: w179 -> [_ w206]
      tunnel: w178 -> [_ w201]
      tunnel: w177 -> [_ w200]
      tunnel: w176 -> [_ w199]
      tunnel: w173 -> [w198 _]
      frame False {
      }
      frame True {
        n117 = Unflatten From String(type=T4."UpdateSubscription", binary string=w206, data includes array or string size? (T)=FALSE) -> (rest of the binary string=w205:string, value=w204:T4)  [unwired: 2 in, 1 out]
        n118 = case shown="\"SubscriptionData\"" w204 {
          tunnel: w208 -> [w211 _ _ _ _]
          tunnel: w205 -> [w220 w258 _ _ _]
          tunnel: w201 -> [_ w260 _ _ _]
          tunnel: w200 -> [_ w261 _ _ _]
          tunnel: w199 -> [_ w259 _ _ _]
          frame "DeviceList" {
            w221 = u8 0  # Number of Devices
            # "struct DeviceList\n{\n    MessageID id;\n    byte NumberOfDevices;\n    DeviceType deviceTypes[];\n    byte deviceIDs[];\n}"
            n119 = Unflatten From String(type=w221, binary string=w220) -> (rest of the binary string=w212:string, value=w217:u8)  [unwired: 3 in, 1 out]
            n120 = for {
              N: w217 -> [_]
              shift-right: [w234] -> _
              shift-left: w212 -> [w236]
              tunnel: [w235] -> w219 mode=indexing
              w237 = u8 0  # DeviceType
              n121 = Unflatten From String(type=w237, binary string=w236) -> (rest of the binary string=w234:string, value=w235:u8)  [unwired: 3 in, 1 out]
            }
            n122 = String Subset(string=w212, offset (0)=w211, length (rest)=w211) -> (substring=w210:string)
            n123 = for {
              N: w217 -> [_]
              shift-right: [w231] -> _
              shift-left: w210 -> [w232]
              tunnel: [w230] -> w218 mode=indexing
              w233 = u8 0  # DeviceID
              n124 = Unflatten From String(type=w233, binary string=w232) -> (rest of the binary string=w231:string, value=w230:u8)  [unwired: 3 in, 1 out]
            }
            n125 = Initialize Array(u8 0, w211, w211) -> (w216:u8[][])
            n126 = for {
              tunnel: w219 -> [w227] mode=indexing
              tunnel: w218 -> [w223] mode=indexing
              shift-right: [w229] -> w213
              shift-left: w216 -> [w225]
              w226 = 0 ("disabled index (col)")
              n127 = Index Array(array=w225, index (row)=w227, index (col)=w226) -> (element=w224:u8)
              n128 = Increment(x=w224) -> (x+1=w222:u8)
              n129 = Replace Array Subset(array=w225, new element=w222, index (row)=w227, index (col)=w226) -> (w228:u8[][])
              n130 = Replace Array Subset(array=w228, new element=w223, index (row)=w227, index (col)=w222) -> (w229:u8[][])
            }
            n131 = control-ref of="DeviceIDs arranged by Type"() -> (w214:refnum<vi>)
            n132 = property class="Arr (strict)"(reference=w214, "Val(Sgnl)"=w213) -> ()  [unwired: 1 in, 2 out]
            n133 = local write "Status"("Recv. DeviceList from JerrysGrapher_RIO" ("Status")) -> ()
          }
          frame "SubscriptionData" {
            n134 = String To Byte Array(string=w258) -> (unsigned byte array=w257:u8[])
            n135 = Get Date/Time In Seconds() -> (seconds since 1Jan1904=w242:timestamp)
            n136 = Delete From Array(array=w257, length=4, index=0) -> (deleted portion=w252:u8[], array with subset deleted=w255:u8[])
            n137 = Reverse 1D Array(array=w252) -> (reversed array=w253:u8[])
            n138 = feedback-in #1(w242) -> ()
            n139 = feedback #1() -> (w241:timestamp)  [unwired: 1 in]
            n140 = Byte Array To String(unsigned byte array=w253) -> (string=w254:string)
            n141 = Subtract(x=w242, y=w241) -> (x-y=w240:dbl)
            n142 = Reshape Array(w255, w261, w260) -> (w250:u8[][])
            n143 = Unflatten From String(type=sgl 0.0, binary string=w254) -> (value=w245:sgl)  [unwired: 3 in, 2 out]
            n144 = Multiply(x=1000.0, y=w240) -> (x*y=→"Real Milliseconds per Packet":dbl)
            n145 = for {
              tunnel: [w280] -> w249 mode=indexing
              tunnel: w250 -> [w278] mode=indexing
              n146 = Reverse 1D Array(array=w278) -> (reversed array=w277:u8[])
              n147 = Type Cast(type=0.0, x=w277) -> (*(type *) &x=w280:dbl)
            }
            n148 = Add(x=w245, y=w259) -> (x+y=w246:timestamp)
            n149 = property on="Plot" class="Clust (strict)"() -> ("Controls[]"=w243:refnum<vi>[])  [unwired: 2 in, 2 out]
            n150 = for {
              tunnel: w243 -> [w269] mode=indexing
              tunnel: w249 -> [w270] mode=indexing
              tunnel: [w274] -> w248 mode=indexing
              tunnel: w246 -> [w273]
              i -> [w276]
              n151 = property class="Ctl"(reference=w269) -> ("Value"=w272:variant)  [unwired: 1 in, 2 out]
              n152 = local read "0"() -> (w268:T1)
              n153 = Variant To Data(type=w268, Variant=w272) -> (data=w267:T1)  [unwired: 1 in, 1 out]
              n154 = Build Array(w270) -> (w275:dbl[])
              n155 = Unbundle By Name(w267) -> ("Y-Axis"=w266:u16, "Plot Color"=w264:u32, "Point Color"=w265:u32)
              n156 = Bundle By Name(cluster=w267, "Current Value"=w270) -> (w271:T1)
              n157 = property on="Waveform chart" class="WFChart (strict)"("Active Plot"=w276) -> (error out=w263:errorcluster)  [unwired: 2 in, 1 out]
              n158 = Bundle By Name("Y"=w275, "t0"=w273) -> (w274:waveform(dbl))  [unwired: 1 in]
              n159 = property class="Ctl"(reference=w269, "Value"=w271) -> ()  [unwired: 1 in, 2 out]
              n160 = property on="Waveform chart" class="WFChart (strict)"(error in=w263, "Plot.Fill/Pt. Color"=w265) -> ()  [unwired: 1 in, 2 out]
              n161 = property on="Waveform chart" class="WFChart (strict)"(error in=w263, "Plot.YScaleIdx"=w266) -> ()  [unwired: 1 in, 2 out]
              n162 = property on="Waveform chart" class="WFChart (strict)"(error in=w263, "Plot.Plot Color"=w264) -> ()  [unwired: 1 in, 2 out]
            }
            n163 = case shown="False" "Stop Data" {
              tunnel: w248 -> [w262 _]
              frame False {
                "Waveform chart" <- w262
              }
              frame True {
              }
            }
          }
          frame Default {
          }
          frame "UpdateSubscription" {
          }
          frame "DeviceListRequest" {
          }
        }
      }
    }
    n164 = Divide(x=1000.0, y=w175) -> (x/y=w172:dbl)
    n165 = feedback #2(0) -> (w187:dbl)
    n166 = Greater Or Equal?(x=w187, y=w172) -> (x >= y?=w174:bool)
    n167 = Multiply(x=w172, y=-10.0) -> (x*y=w170:dbl)
    n168 = feedback #3(1) -> (w185:i32)
    n169 = case shown="True" w174 {
      tunnel: [w282 w287] -> w188
      tunnel: w187 -> [w283 _]
      tunnel: w185 -> [w281 w294]
      tunnel: [w281 w293] -> w184
      tunnel: w183 -> [_ w292]
      tunnel: w182 -> [_ w290]
      tunnel: w181 -> [_ w289]
      tunnel: w173 -> [_ w285]
      tunnel: w170 -> [_ w284]
      frame False {
        n170 = Increment(x=w283) -> (x+1=w282:dbl)
      }
      frame True {
        # "struct DeviceListRequest\n{\n    MessageID id;\n}"
        n171 = Select(t=0, s=w285, f=w284) -> (s? t:f=w287:dbl)
        n172 = Increment(x=w294) -> (x+1=w293:i32)
        n173 = Number To Decimal String(number=w294) -> (decimal integer string=w298:string)  [unwired: 1 in]
        n174 = Concatenate Strings("Sending Inital Handshake (" ("string"), w298, "th time)" ("string")) -> (w295:string)
        n175 = local write "Status"(w295) -> ()
        n176 = Flatten To String(anything=T4."DeviceListRequest") -> (data string=w291:string)  [unwired: 3 in, 2 out]
        n177 = UDP Write(address=w290, port or service name=w289, connection ID=w292, data in=w291) -> ()  [unwired: 2 in, 2 out]
      }
    }
    n178 = feedback-in #2(w188) -> ()
    n179 = feedback-in #3(w184) -> ()
  }
